vi "Day 15-Calculate Score.vi"(7 "Risk":i32[][](array[numeric]), 8 "G":i32[][](array[numeric]), 9 "Neighbor":T1, 10 "Current":T1, 11 "Goal":T1) -> (2 "gScore(neighbor)":i32, 3 "fScore(neighbor)":i32)   [LabVIEW 2021]
uses:
  Day 15-Position.ctl
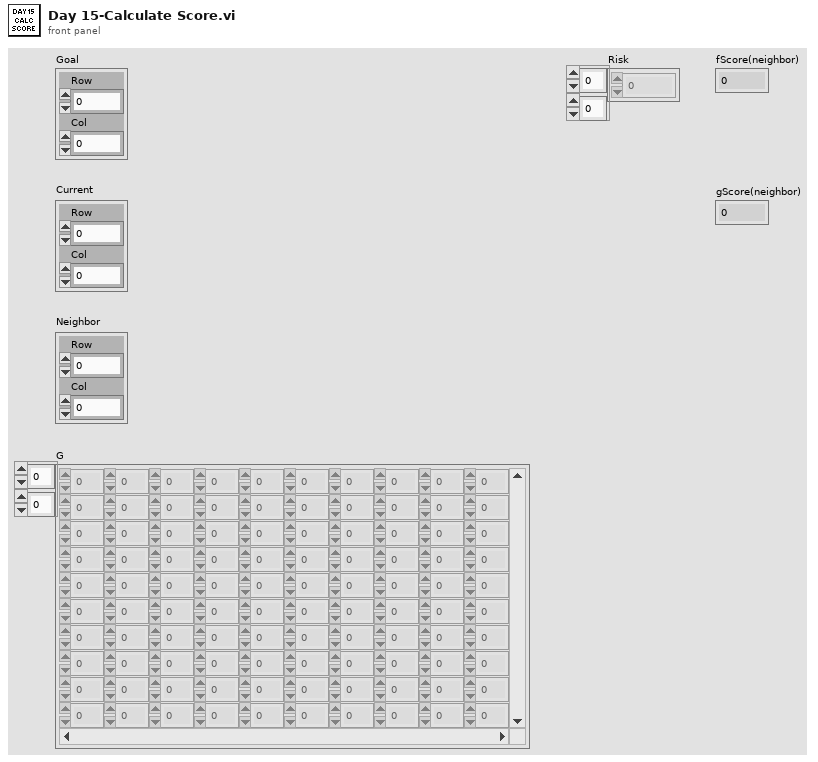
[diagram p1: front panel]
types:
  T1 = typedef "Day 15-Position.ctl" = cluster{"Row":i32, "Col":i32}
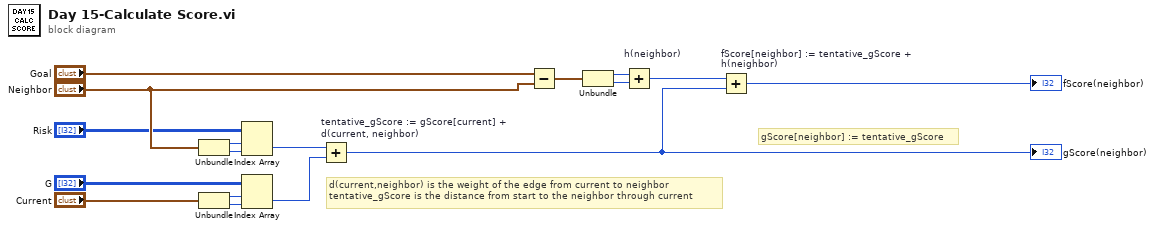
[diagram p0: block diagram]
diagram:
  # "gScore[neighbor] := tentative_gScore"
  # "d(current,neighbor) is the weight of the edge from current to neighbor\ntentative_gScore is the distance from start to the neighbor through current"
  n1 = Unbundle("Neighbor") -> ("Row"=w17:i32, "Col"=w16:i32)
  n2 = Unbundle("Current") -> ("Row"=w7:i32, "Col"=w6:i32)
  n3 = Index Array(array="Risk", index (row)=w17, index (col)=w16) -> (element=w15:i32)
  n4 = Index Array(array="G", index (row)=w7, index (col)=w6) -> (element=w4:i32)
  n5 = Add "tentative_gScore := gScore[current] + d(current, neighbor)"(x=w15, y=w4) -> (x+y=w9:i32)
  "gScore(neighbor)" <- w9
  n6 = Subtract(x="Goal", y="Neighbor") -> (x-y=w13:T1)
  n7 = Unbundle(w13) -> ("Row"=w12:i32, "Col"=w11:i32)
  n8 = Add "h(neighbor)"(x=w12, y=w11) -> (x+y=w10:i32)
  n9 = Add "fScore[neighbor] := tentative_gScore + h(neighbor)"(x=w10, y=w9) -> (x+y=→"fScore(neighbor)":i32)
